vi "Server.vi"() -> ()   [LabVIEW 2019]
uses:
  <vilib>/Utility/file.llb/Write Delimited Spreadsheet (string).vi
  <vilib>/Utility/file.llb/Read Delimited Spreadsheet (string).vi
  <vilib>/regexp/Match Regular Expression.xnode
panel:
  out "History":string[][](table)
  out "Status":string
  out "START LED":bool
  in  "START":bool
  # "Car Wash Server"
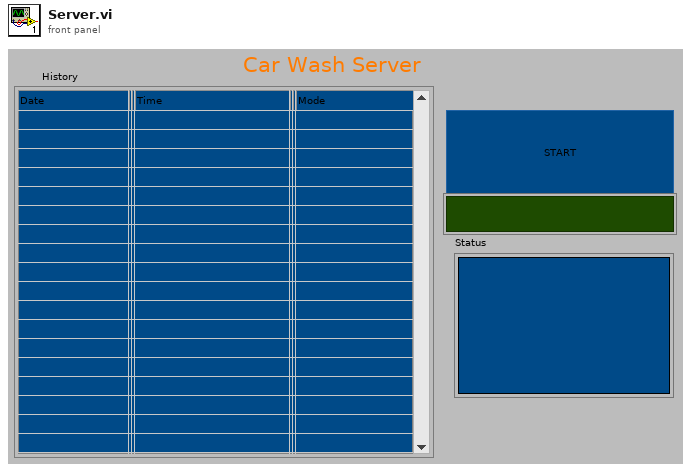
[diagram p1: front panel]
types:
  T1 = enum8{"Enabled", "Disabled", "Disabled and Grayed Out"}
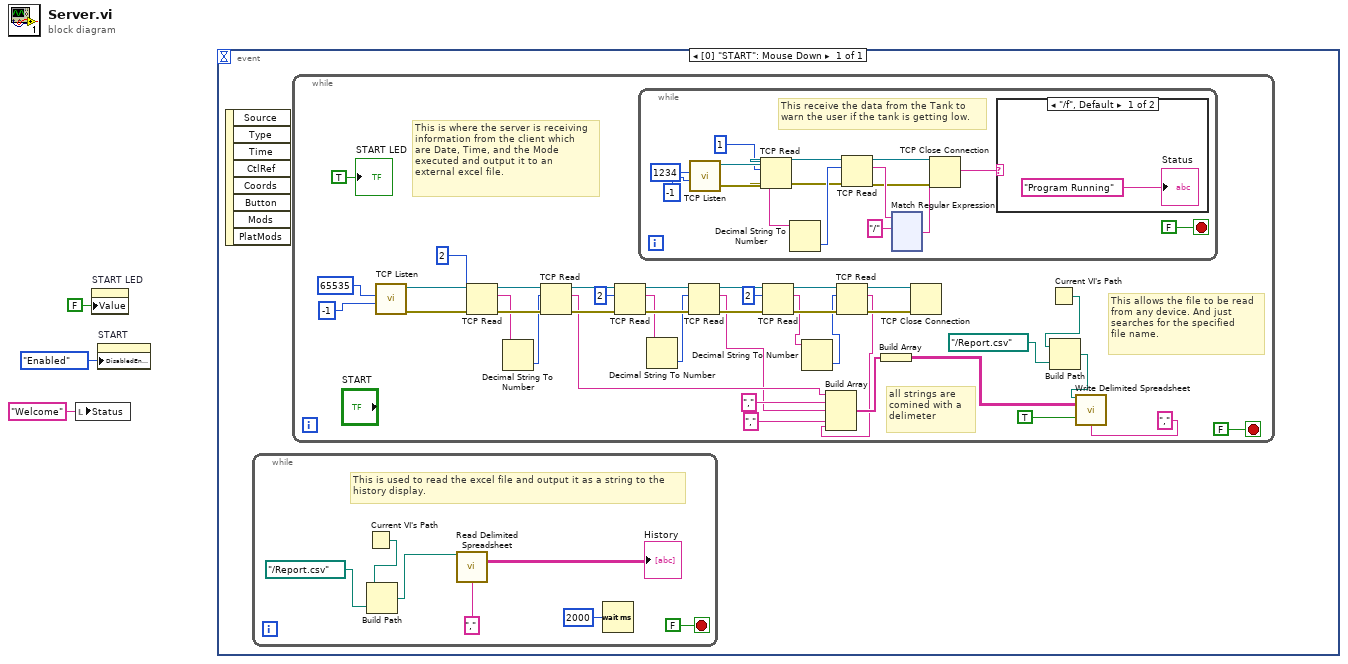
[diagram p0: block diagram]
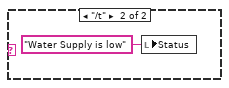
[diagram p2: hidden frame]
diagram:
  n1 = local write "Status"("Welcome" ("Status")) -> ()
  n2 = property on="START LED" class="Bool (strict)"("Value"=FALSE ("START LED")) -> ()  [unwired: 2 in, 2 out]
  n3 = property on="START" class="Bool (strict)"("DisabledEnum"=T1."Enabled" ("Disabled")) -> ()  [unwired: 2 in, 2 out]
  n4 = event shown="[0] \"START\": Mouse Down" {
    selector: _ -> [_]
    dyn-events: _ -> [_]
    timeout: _ -> [_]
    event "START": Mouse Down {
      n5 = event-data() -> ()  [unwired: 1 in, 8 out]
      n6 = while {
        stop <- FALSE stop-if-true
        # "This is used to read the excel file and output it as a string to the\nhistory display."
        n7 = Current VI's Path() -> (path=w5:path)
        n8 = Build Path(base path=w5, name or relative path=path "../Report.csv" ("base path")) -> (appended path=w6:path)
        n9 = call-poly <vilib>:"Read Delimited Spreadsheet.vi"("file path (dialog if empty)"=w6, "delimiter (\\t)"="," ("delimiter (\\t)")) -> ("all rows"=→"History":string[][])  [unwired: 8 in, 5 out]
        n10 = Wait (ms)(milliseconds to wait=u32 2000) -> ()  [unwired: 1 out]
      }
      n11 = while {
        stop <- FALSE stop-if-true
        # "This allows the file to be read\nfrom any device. And just\nsearches for the specified \nfile name."
        # "all strings are \ncomined with a \ndelimeter"
        # "This is where the server is receiving\ninformation from the client which \nare Date, Time, and the Mode\nexecuted and output it to an \nexternal excel file."
        n12 = call <vilib>:"TCP Listen.vi"("timeout ms (wait forever: -1)"=-1, "port"=u16 65535) -> ("error out"=w48:errorcluster, "connection ID"=w39:refnum<k5>)  [unwired: 5 in, 3 out]
        n13 = TCP Read(connection ID=w39, bytes to read=2, error in (no error)=w48) -> (connection ID out=w38:refnum<k5>, data out=w34:string, error out=w47:errorcluster)  [unwired: 2 in]
        n14 = Decimal String To Number(string=w34) -> (number=w33:i32)  [unwired: 2 in, 1 out]
        n15 = TCP Read(connection ID=w38, bytes to read=w33, error in (no error)=w47) -> (connection ID out=w37:refnum<k5>, data out=w18:string, error out=w46:errorcluster)  [unwired: 2 in]
        n16 = TCP Read(connection ID=w37, bytes to read=2, error in (no error)=w46) -> (connection ID out=w36:refnum<k5>, data out=w29:string, error out=w45:errorcluster)  [unwired: 2 in]
        n17 = while {
          stop <- FALSE stop-if-true
          # "This receive the data from the Tank to\nwarn the user if the tank is getting low."
          n18 = call <vilib>:"TCP Listen.vi"("timeout ms (wait forever: -1)"=-1, "port"=u16 1234) -> ("error out"=w61:errorcluster, "connection ID"=w56:refnum<k5>)  [unwired: 5 in, 3 out]
          n19 = TCP Read(connection ID=w56, bytes to read=1, error in (no error)=w61) -> (connection ID out=w57:refnum<k5>, data out=w62:string, error out=w60:errorcluster)  [unwired: 2 in]
          n20 = Decimal String To Number(string=w62) -> (number=w63:i32)  [unwired: 2 in, 1 out]
          n21 = TCP Read(connection ID=w57, bytes to read=w63, error in (no error)=w60) -> (connection ID out=w58:refnum<k5>, data out=w64:string, error out=w59:errorcluster)  [unwired: 2 in]
          n22 = xnode "Match Regular Expression"("input string"=w64, "regular expression"="/") -> ("after match"=w50:string)  [unwired: 4 in, 4 out]
          n23 = TCP Close Connection(connection ID=w58, error in (no error)=w59) -> ()  [unwired: 1 in, 2 out]
          n24 = case shown="\"/f\", Default" w50 {
            frame "/f", Default {
              "Status" <- "Program Running" ("String")
            }
            frame "/t" {
              n25 = local write "Status"("Water Supply is low" ("Status")) -> ()
            }
          }
        }
        n26 = Decimal String To Number(string=w29) -> (number=w28:i32)  [unwired: 2 in, 1 out]
        n27 = TCP Read(connection ID=w36, bytes to read=w28, error in (no error)=w45) -> (connection ID out=w35:refnum<k5>, data out=w17:string, error out=w44:errorcluster)  [unwired: 2 in]
        n28 = TCP Read(connection ID=w35, bytes to read=2, error in (no error)=w44) -> (connection ID out=w40:refnum<k5>, data out=w27:string, error out=w43:errorcluster)  [unwired: 2 in]
        n29 = Decimal String To Number(string=w27) -> (number=w26:i32)  [unwired: 2 in, 1 out]
        n30 = TCP Read(connection ID=w40, bytes to read=w26, error in (no error)=w43) -> (connection ID out=w41:refnum<k5>, data out=w16:string, error out=w42:errorcluster)  [unwired: 2 in]
        n31 = Build Array "Build Array"(w18, "," ("element"), w17, "," ("element"), w16) -> (w22:string[])
        n32 = Build Array(w22) -> (w19:string[][])
        n33 = TCP Close Connection(connection ID=w41, error in (no error)=w42) -> ()  [unwired: 1 in, 2 out]
        n34 = Current VI's Path() -> (path=w13:path)
        n35 = Build Path(base path=w13, name or relative path=path "../Report.csv" ("base path")) -> (appended path=w12:path)
        n36 = call-poly <vilib>:"Write Delimited Spreadsheet.vi"("file path (dialog if empty)"=w12, "2D data"=w19, "append to file? (new file:F)"=TRUE, "delimiter (\\t)"="," ("delimiter (\\t)")) -> ()  [unwired: 10 in, 2 out]
        "START LED" <- TRUE ("START LED")
      }
    }
  }
